vi "FT_Get_Device_Info.vi"(0 "Handle":u32) -> (1 "FT_Status":u32, 2 "Device Information":T1)   [LabVIEW 2011]
uses:
  FTD2XX.dll
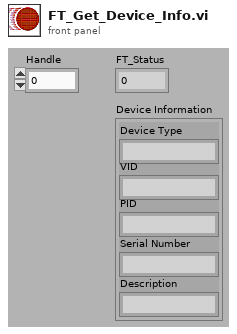
[diagram p1: front panel]
types:
  T1 = cluster{"Device Type":string, "VID":string, "PID":string, "Serial Number":string, "Description":string}
  T2 = cluster{string, string, string, "SerialNumber":string, "Description":string}
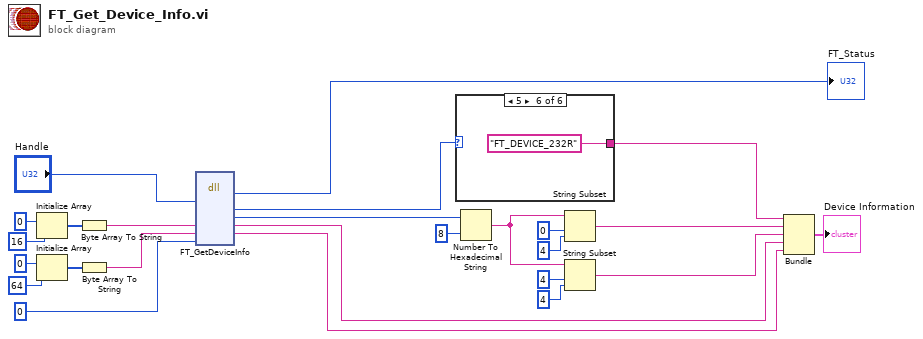
[diagram p0: block diagram]
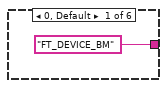
[diagram p2: hidden frame]
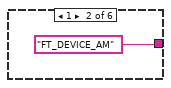
[diagram p3: hidden frame]
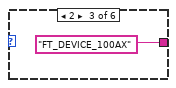
[diagram p4: hidden frame]
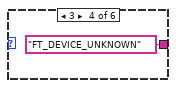
[diagram p5: hidden frame]
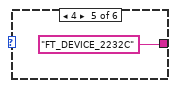
[diagram p6: hidden frame]
diagram:
  n1 = Initialize Array(u8 0, 16 ("dimension size")) -> (w7:u8[])
  n2 = Initialize Array(u8 0, 64 ("dimension size")) -> (w5:u8[])
  n3 = Byte Array To String(unsigned byte array=w7) -> (string=w1:string)
  n4 = Byte Array To String(unsigned byte array=w5) -> (string=w2:string)
  n5 = dll-call lib="C:/Work/Labview/#Avesta/D2XX_Functions_7.0/FTD2XX.dll" fn="FT_GetDeviceInfo"("Handle"="Handle", "SerialNumber"=w1, "Description"=w2, "Dummy"=u32 0) -> ("FT_Status"=→"FT_Status":u32, "DeviceType"=w16:u32, "ID"=w23:u32, "SerialNumber"=w12:string, "Description"=w11:string)  [unwired: 4 in, 5 out]
  n6 = case shown="5" w16 {
    tunnel: ["FT_DEVICE_BM" "FT_DEVICE_AM" "FT_DEVICE_100AX" "FT_DEVICE_UNKNOWN" "FT_DEVICE_2232C" "FT_DEVICE_232R"] -> w15
    frame 0, Default {
    }
    frame 1 {
    }
    frame 2 {
    }
    frame 3 {
    }
    frame 4 {
    }
    frame 5 {
    }
  }
  n7 = Number To Hexadecimal String(1:i16 8 ("width (-)"), 2:w23) -> (0:w17:string)
  n8 = String Subset(string=w17, offset (0)=0, length (rest)=4 ("length (rest)")) -> (substring=w14:string)
  n9 = String Subset(string=w17, offset (0)=4, length (rest)=4 ("length (rest)")) -> (substring=w13:string)
  n10 = Bundle(w15, w14, w13, "SerialNumber"=w12, "Description"=w11) -> (→"Device Information":T2)  [unwired: 1 out]
